vi "TCP Receive Message.vi"(8 "error in (no error)":errorcluster, 9 "timeout [ms]":i32=1000, 11 "TCP Connection in":refnum<k5>) -> (0 "error out":errorcluster, 1 "Flattened Payload":string, 2 "Message Type":T1, 3 "TCP Connection out":refnum<k5>, 4 "Received Bytes":i32)   [LabVIEW 2020, in "hse-network.lvlib"]
doc: "____\nHAMPEL SOFTWARE ENGINEERING v3.8.0 (2023-12-18 14:41)"
uses:
  hse-network.lvlib
  Message Types Enum.ctl
  TCP Message.ctl
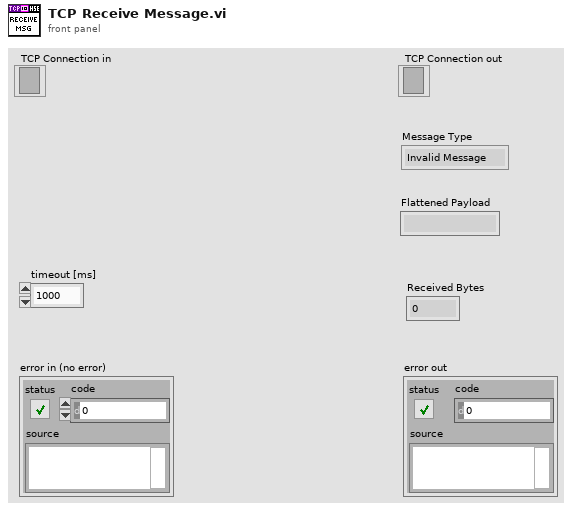
[diagram p1: front panel]
types:
  T1 = typedef "hse-network.lvlib/Message Types Enum.ctl" = enum8{"Invalid Message", "Check-Message", "MHL-Command", "String", "1D-Array Wfm", "2D-Array DBL", "2D-Array I32"}
  T2 = typedef "hse-network.lvlib/TCP Message.ctl" = cluster{"Message Type":T1, "Flattened Payload":string, "Client Error":errorcluster}
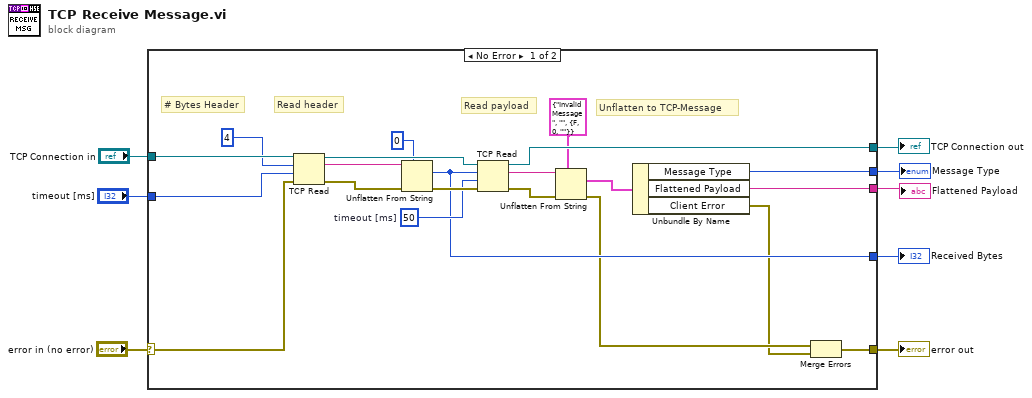
[diagram p0: block diagram]
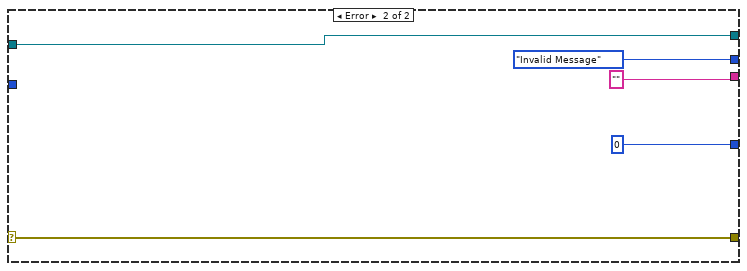
[diagram p2: hidden frame]
diagram:
  n1 = case shown="No Error" "error in (no error)" {
    selector: "error in (no error)" -> [w22 w34]
    tunnel: [w29 w32] -> w8
    tunnel: "TCP Connection in" -> [w26 w32]
    tunnel: [w18 0 ("blocksize")] -> w6
    tunnel: [w10 w34] -> w5
    tunnel: "timeout [ms]" -> [w21 _]
    tunnel: [w12 Message_Types_Enum."Invalid Message" ("Message Type")] -> w2
    tunnel: [w11 "" ("Flattened Payload")] -> w1
    frame No Error {
      w19 = 50  # timeout [ms]
      # "Unflatten to TCP-Message"
      # "# Bytes Header"
      # "Read payload"
      # "Read header"
      n2 = TCP Read(connection ID=w26, bytes to read=4, error in (no error)=w22, 9:w21) -> (connection ID out=w24:refnum<k5>, data out=w20:string, error out=w27:errorcluster)  [unwired: 1 in]
      n3 = Unflatten From String(type=0 ("blocksize"), binary string=w20, error in (no error)=w27) -> (value=w18:i32, error out=w28:errorcluster)  [unwired: 2 in, 1 out]
      n4 = TCP Read(connection ID=w24, bytes to read=w18, error in (no error)=w28, 9:w19) -> (connection ID out=w29:refnum<k5>, data out=w16:string, error out=w17:errorcluster)  [unwired: 1 in]
      n5 = Unflatten From String(type=T2 {"Message Type"=enum."Invalid Message", "Flattened Payload"="", "Client Error"={"status"=FALSE, "code"=0, "source"=""}} ("TCP Message"), binary string=w16, error in (no error)=w17) -> (value=w13:T2, error out=w14:errorcluster)  [unwired: 2 in, 1 out]
      n6 = Unbundle By Name(w13) -> ("Message Type"=w12:T1, "Flattened Payload"=w11:string, "Client Error"=w9:errorcluster)
      n7 = Merge Errors(w14, w9) -> (w10:errorcluster)
    }
    frame Error {
    }
  }
  "TCP Connection out" <- w8
  "error out" <- w5
  "Received Bytes" <- w6
  "Message Type" <- w2
  "Flattened Payload" <- w1
